vi "write muxlist to top.vi"(8 "error in (no error)":errorcluster, 10 "MuxList":cluster{"Src":string, "Dests":string[]}[](array[cluster]), 11 "Refnum in":T1) -> (0 "error out":errorcluster, 3 "Refnum out":T1)   [LabVIEW 2015, in "SLSC Switch.lvlib" / "SLSC Switch.lvclass"]
uses:
  SLSC Switch.lvclass
  <vilib>/Utility/config.llb/Config Data RefNum.ctl
  <vilib>/Utility/config.llb/Write Key (String).vi
  <vilib>/Utility/config.llb/NI_LVConfig.lvlib
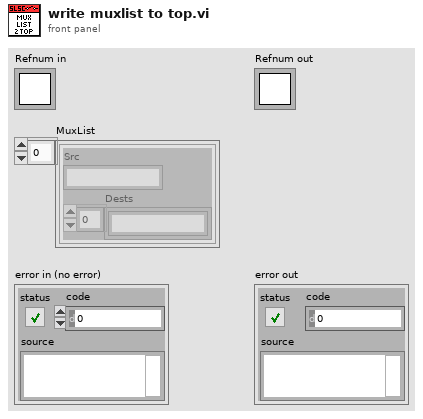
[diagram p1: front panel]
types:
  T1 = typedef "NI_LVConfig.lvlib/Config Data RefNum.ctl" = refnum<k1>
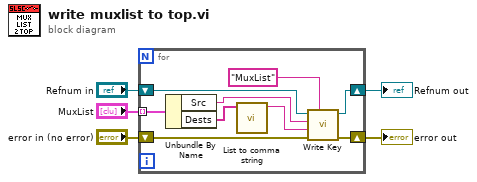
[diagram p0: block diagram]
diagram:
  n1 = for {
    shift-right: [w13] -> w4
    shift-left: "error in (no error)" -> [w14]
    tunnel: "MuxList" -> [w6] mode=indexing
    shift-right: [w11] -> w2
    shift-left: "Refnum in" -> [w12]
    n2 = Unbundle By Name(w6) -> ("Src"=w8:string, "Dests"=w9:string[])
    n3 = call "List to comma string.vi"("Array"=w9) -> ("String"=w7:string)  [unwired: 10 in]
    n4 = call-poly <vilib>:"Write Key.vi"("section"="MuxList", "error in (no error)"=w14, "value"=w7, "key"=w8, "refnum"=w12) -> ("error out"=w13:errorcluster, "refnum out"=w11:T1)  [unwired: 4 in, 1 out]
  }
  "error out" <- w4
  "Refnum out" <- w2
